vi "UNIX-DATE_TIME.vi"(2 "TIME_BASE":u32, 3 "FRACSEC":u64, 4 "SOC":u64) -> (0 "Date/Time":string, 1 "seconds":dbl)   [LabVIEW 2013]
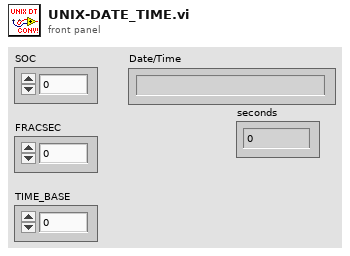
[diagram p1: front panel]
types:
  T1 = typedef "LVDateTimeRec.ctl" = cluster{"fractional second":dbl, "second":i32, "minute":i32, "hour":i32, "day of month":i32, "month":i32, "year":i32, "day of week":i32, "day of year":i32, "DST":i32}
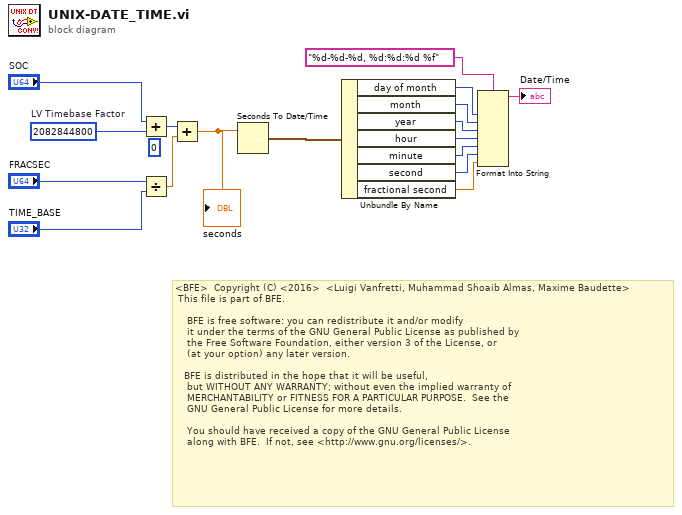
[diagram p0: block diagram]
diagram:
  (unwired) u64 0 ("y")
  w3 = u64 2082844800  # LV Timebase Factor
  # "<BFE>  Copyright (C) <2016>  <Luigi Vanfretti, Muhammad Shoaib Almas, Maxime Baudette>\n This file is part of BFE.\n\n    BFE is free software: you can redistribute it and/or modify\n    it under the terms of the GNU General Public License as published by\n    the Free Software Foundation, either version 3 of the License, or\n    (at your option) any later version.\n\n   BFE is distributed in the hope that it will be useful,\n    but WITHOUT ANY WARRANTY; without even the implied warranty of\n    MERCHANTABILITY or FITNESS FOR A PARTICULAR PURPOSE.  See the\n    GNU General Public License for more details.\n\n    You should have received a copy of the GNU General Public License\n    along with BFE.  If not, see <http://www.gnu.org/licenses/>."
  n1 = Add(x="SOC", y=w3) -> (x+y=w15:u64)
  n2 = Divide(x="FRACSEC", y="TIME_BASE") -> (x/y=w2:dbl)
  n3 = Add(x=w15, y=w2) -> (x+y=w16:dbl)
  "seconds" <- w16
  n4 = Seconds To Date/Time(time stamp (now)=w16) -> (date time rec=w5:T1)  [unwired: 1 in]
  n5 = Unbundle By Name(w5) -> ("day of month"=w6:i32, "month"=w7:i32, "year"=w8:i32, "hour"=w9:i32, "minute"=w10:i32, "second"=w11:i32, "fractional second"=w1:dbl)
  n6 = Format Into String(format string="%d-%d-%d, %d:%d:%d %f", w6, w7, w8, w9, w10, w11, w1) -> (resulting string=→"Date/Time":string)  [unwired: 2 in, 1 out]
